vi "DIO Timing Test.vi"() -> ()   [LabVIEW 2020]
uses:
  <vilib>/DAQmx/write.llb/DAQmx Write (Digital Bool 1Line 1Point).vi
  9abfa4c0-cf51-4809-8978-549f57bc71e0.vi
  68ffd5a6-70b5-4e5e-b21d-805be59154c4.vi
  Utility VIs/Controls/Utilities-Wait.vi/89bc9713-8f2c-40bd-a11f-1c800a437687.vi
  <vilib>/Utility/High Resolution Relative Seconds.vi
  <vilib>/DAQmx/create/channels.llb/DAQmx Create Channel (DO-Digital Output).vi
  <vilib>/Utility/High Resolution Polling Wait.vi
  <vilib>/DAQmx/miscellaneous.llb/DAQmx Fill In Error Info.vi
  <vilib>/gmath/NI_Gmath.lvlib
  <vilib>/DAQmx/create/channels.llb/DAQmx Create Channel (DI-Digital Input).vi
  <vilib>/DAQmx/read.llb/DAQmx Read (Digital Bool 1Line 1Point).vi
panel:
  out "Graph":dbl[](graph)
  out "median":dbl format="%.3f ms"
  out "timing":T1(graph)
  out "Iteration":i32
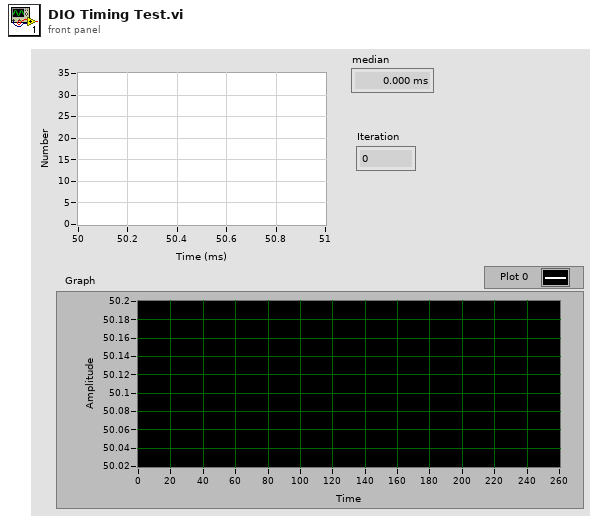
[diagram p1: front panel]
types:
  T1 = cluster{"X Values":dbl[], "Histogram: h(x)":i32[]}
  T2 = enum16{"arithmetic", "geometric", "harmonic", "trimmed", "median"}
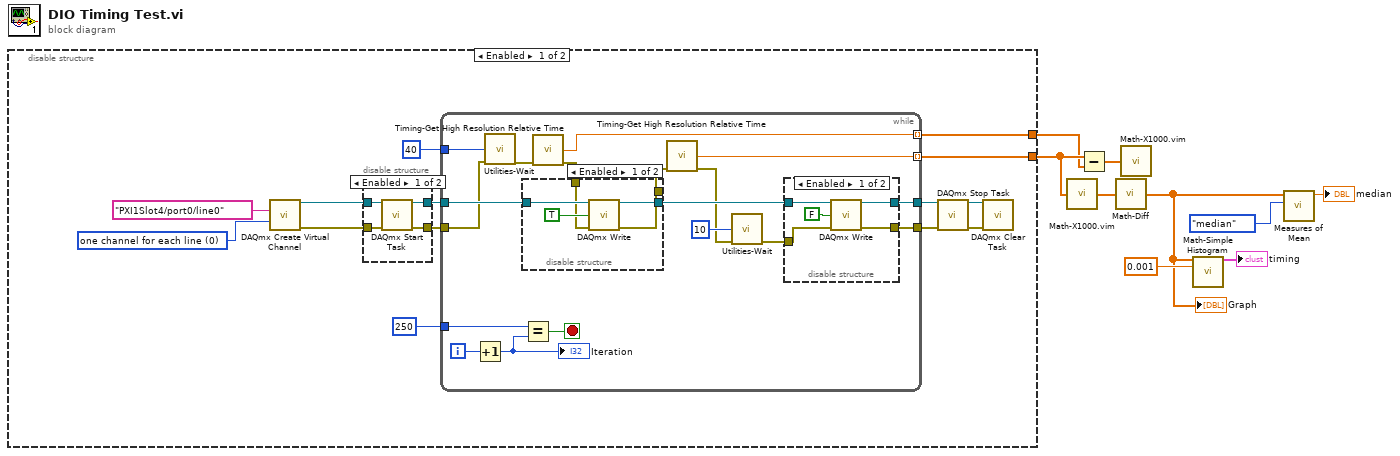
[diagram p0: block diagram]
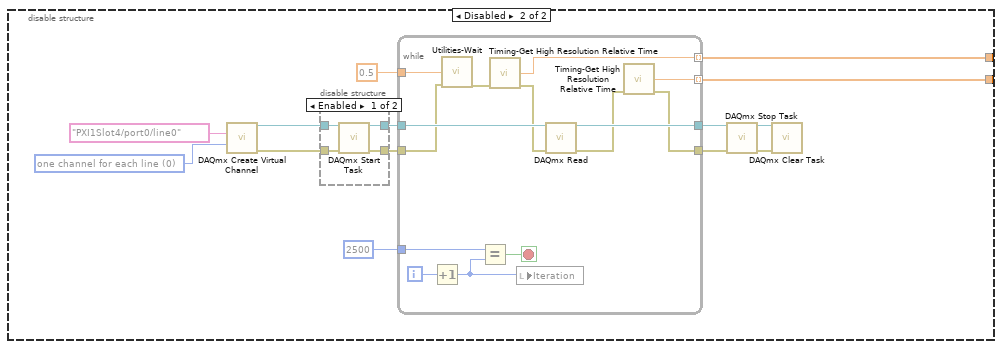
[diagram p5: hidden frame]
diagram:
  n1 = disable-structure shown="Enabled" {
    disable-tunnel: [w15 w67] -> w5
    disable-tunnel: [w14 w66] -> w4
    frame Enabled {
      w22 = 0 items=["one channel for each line", "one channel for all lines"] ("line grouping")
      n2 = call-poly <vilib>:"DAQmx Create Virtual Channel.vi"("lines"=tag "PXI1Slot4/port0/line0", "line grouping"=w22) -> ("task out"=w11:refnum<k21>, "error out"=w10:errorcluster)  [unwired: 12 in]
      n3 = disable-structure shown="Enabled" {
        disable-tunnel: [w27 w29] -> w13
        disable-tunnel: [w26 w28] -> w12
        disable-tunnel: w11 -> [w25 w29]
        disable-tunnel: w10 -> [w24 w28]
        frame Enabled {
          n4 = call <vilib>:"DAQmx Start Task.vi"("task/channels in"=w25, "error in"=w24) -> ("task out"=w27:refnum<k21>, "error out"=w26:errorcluster)  [unwired: 12 in]
        }
        frame Disabled {
        }
      }
      n5 = while {
        tunnel: w13 -> [w47]
        tunnel: [w43] -> w19
        tunnel: [w42] -> w18
        tunnel: [w40] -> w15 mode=indexing
        tunnel: 250 ("x") -> [w41]
        tunnel: u32 40 ("milliseconds to wait") -> [w39]
        tunnel: w12 -> [w38]
        tunnel: [w30] -> w14 mode=indexing
        i -> [w34]
        stop <- w35 stop-if-true
        n6 = Increment(x=w34) -> (x+1=w33:i32)
        "Iteration" <- w33
        n7 = call "Utilities-Wait.vi"("milliseconds to wait"=w39, "error in (no error)"=w38) -> ("error out"=w32:errorcluster)  [unwired: 13 in]
        n8 = Equal?(x=w41, y=w33) -> (x = y?=w35:bool)
        n9 = call "Timing-Get High Resolution Relative Time.vi"("error in (no error)"=w32) -> ("double precision float"=w30:dbl, "error out"=w31:errorcluster)  [unwired: 13 in]
        n10 = disable-structure shown="Enabled" {
          disable-tunnel: w47 -> [w59 w60]
          disable-tunnel: [w58 w60] -> w45
          disable-tunnel: [w57 w61] -> w37
          disable-tunnel: w31 -> [w55 w61]
          frame Enabled {
            n11 = call-poly <vilib>:"DAQmx Write.vi"("task/channels in"=w59, "data"=TRUE, "error in"=w55) -> ("task out"=w58:refnum<k21>, "error out"=w57:errorcluster)  [unwired: 10 in, 1 out]
          }
          frame Disabled {
          }
        }
        n12 = call "Timing-Get High Resolution Relative Time.vi"("error in (no error)"=w37) -> ("double precision float"=w40:dbl, "error out"=w36:errorcluster)  [unwired: 13 in]
        n13 = call "Utilities-Wait.vi"("milliseconds to wait"=u32 10, "error in (no error)"=w36) -> ("error out"=w44:errorcluster)  [unwired: 13 in]
        n14 = disable-structure shown="Enabled" {
          disable-tunnel: w45 -> [w52 w54]
          disable-tunnel: w44 -> [w51 w53]
          disable-tunnel: [w50 w54] -> w43
          disable-tunnel: [w49 w53] -> w42
          frame Enabled {
            n15 = call-poly <vilib>:"DAQmx Write.vi"("task/channels in"=w52, "data"=FALSE, "error in"=w51) -> ("task out"=w50:refnum<k21>, "error out"=w49:errorcluster)  [unwired: 10 in, 1 out]
          }
          frame Disabled {
          }
        }
      }
      n16 = call <vilib>:"DAQmx Stop Task.vi"("task/channels in"=w19, "error in"=w18) -> ("task out"=w21:refnum<k21>, "error out"=w20:errorcluster)  [unwired: 12 in]
      n17 = call <vilib>:"DAQmx Clear Task.vi"("task in"=w21, "error in"=w20) -> ()  [unwired: 13 in, 1 out]
    }
    frame Disabled {
      w74 = 0 items=["one channel for each line", "one channel for all lines"] ("line grouping")
      n18 = call-poly <vilib>:"DAQmx Create Virtual Channel.vi"("lines"=tag "PXI1Slot4/port0/line0", "line grouping"=w74) -> ("task out"=w63:refnum<k21>, "error out"=w62:errorcluster)  [unwired: 12 in]
      n19 = disable-structure shown="Enabled" {
        disable-tunnel: [w79 w81] -> w65
        disable-tunnel: [w78 w80] -> w64
        disable-tunnel: w63 -> [w77 w81]
        disable-tunnel: w62 -> [w76 w80]
        frame Enabled {
          n20 = call <vilib>:"DAQmx Start Task.vi"("task/channels in"=w77, "error in"=w76) -> ("task out"=w79:refnum<k21>, "error out"=w78:errorcluster)  [unwired: 12 in]
        }
        frame Disabled {
        }
      }
      n21 = while {
        tunnel: w65 -> [w95]
        tunnel: [w94] -> w71
        tunnel: [w88] -> w70
        tunnel: [w92] -> w67 mode=indexing
        tunnel: 2500 ("x") -> [w93]
        tunnel: 0.5 ("milliseconds to wait") -> [w91]
        tunnel: w64 -> [w90]
        tunnel: [w83] -> w66 mode=indexing
        i -> [w86]
        stop <- w87 stop-if-true
        n22 = Increment(x=w86) -> (x+1=w82:i32)
        n23 = call "Utilities-Wait.vi"("milliseconds to wait"=w91, "error in (no error)"=w90) -> ("error out"=w85:errorcluster)  [unwired: 13 in]
        n24 = Equal?(x=w93, y=w82) -> (x = y?=w87:bool)
        n25 = call "Timing-Get High Resolution Relative Time.vi"("error in (no error)"=w85) -> ("double precision float"=w83:dbl, "error out"=w84:errorcluster)  [unwired: 13 in]
        n26 = local write "Iteration"(w82) -> ()
        n27 = call-poly <vilib>:"DAQmx Read.vi"("task/channels in"=w95, "error in"=w84) -> ("task out"=w94:refnum<k21>, "error out"=w89:errorcluster)  [unwired: 11 in, 1 out]
        n28 = call "Timing-Get High Resolution Relative Time.vi"("error in (no error)"=w89) -> ("double precision float"=w92:dbl, "error out"=w88:errorcluster)  [unwired: 13 in]
      }
      n29 = call <vilib>:"DAQmx Stop Task.vi"("task/channels in"=w71, "error in"=w70) -> ("task out"=w73:refnum<k21>, "error out"=w72:errorcluster)  [unwired: 12 in]
      n30 = call <vilib>:"DAQmx Clear Task.vi"("task in"=w73, "error in"=w72) -> ()  [unwired: 13 in, 1 out]
    }
  }
  n31 = call "Math-X1000.vim"("X"=w5) -> ("1000X"=w3:dbl[])
  n32 = Subtract(x=w5, y=w4) -> (x-y=w2:dbl[])
  n33 = call "Math-Diff.vi"("X"=w3) -> ("diff(X)"=w1:dbl[])
  "Graph" <- w1
  n34 = call "Math-X1000.vim"("X"=w2) -> ()  [unwired: 1 out]
  n35 = call "Math-Simple Histogram.vi"("Array"=w1, "Binwidth"=0.001 ("Step")) -> ("Histogram Graph"=→"timing":T1)  [unwired: 13 in]
  n36 = call <vilib>:"Measures of Mean.vi"("type"=T2."median", "x array"=w1) -> ("mean value"=→"median":dbl)  [unwired: 8 in, 1 out]
